vi "Setup TS DAC.vi"(8 "error in":errorcluster, 11 "HTS Test Stand in":refnum<class "HTS Test Stand.lvclass">) -> (0 "error out":errorcluster, 3 "HTS Test Stand out":refnum<class "HTS Test Stand.lvclass">)   [LabVIEW 2019, in "Test Stands.lvlib" / "HTS Test Stand.lvclass"]
uses:
  HTS Test Stand.lvclass
  C:/Users/wg/Documents/LV_Projects/test-stand/App/Generic Test Stand/Generic Test Stand.lvclass
  DAC/LNG Boiling/Heater Box Temperatures/DAC Heater Box Temperatures.lvclass
  C:/Users/wg/Documents/LV_Projects/test-stand/App/DAC/DAC.lvclass
  DAC/DAC.lvclass
  DAC/LNG Boiling/Shunt dU/DAC Shunt dU.lvclass
  DAC/LNG Boiling/Heater dU/DAC Heater dU.lvclass
  DAC/LNG Boiling/Heater Ctrl/DAC Heater Ctrl.lvclass
  DAC/DAC.lvclass/DAC.ctl
  Generic Test Stand/Generic Test Stand.lvclass/Generic Test Stand.ctl
  Generic Test Stand/Generic Test Stand.lvclass
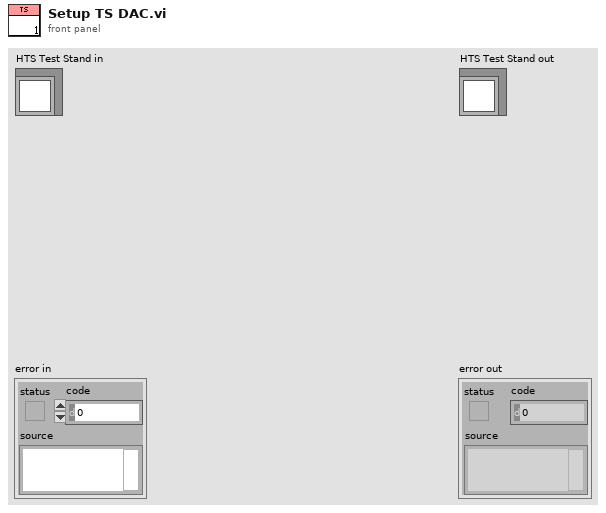
[diagram p1: front panel]
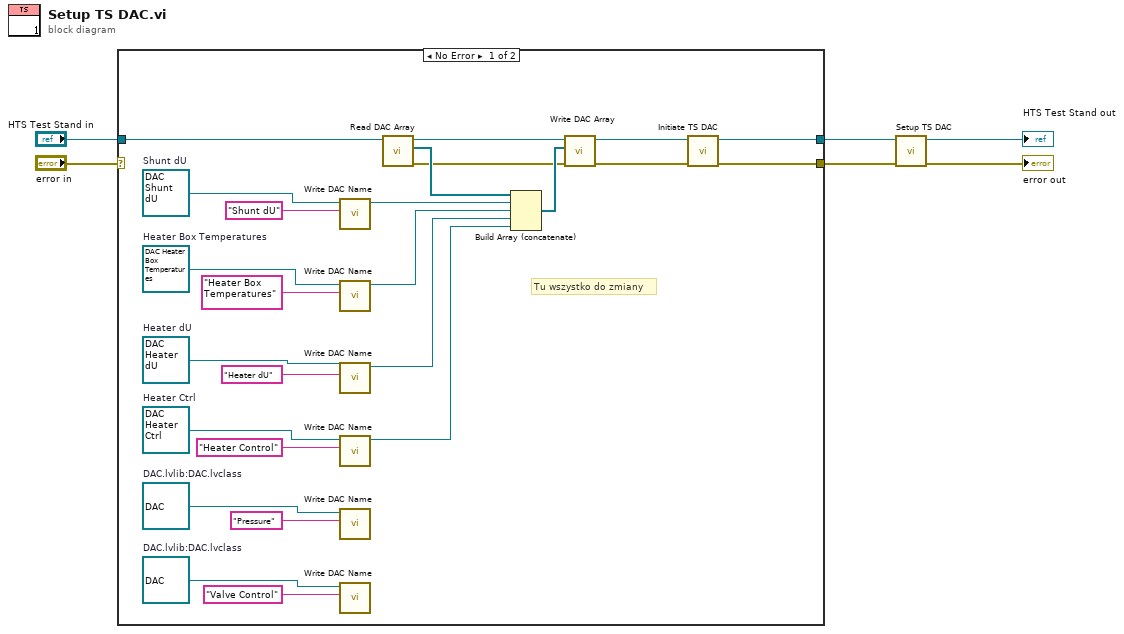
[diagram p0: block diagram]
diagram:
  n1 = case shown="No Error" "error in" {
    selector: "error in" -> [_ w32]
    tunnel: "HTS Test Stand in" -> [w26 w33]
    tunnel: [w8 w33] -> w2
    tunnel: [w7 w32] -> w1
    frame No Error {
      w11 = refnum<class "DAC Heater Ctrl.lvclass"> refnum  # Heater Ctrl
      w13 = refnum<class "DAC Heater dU.lvclass"> refnum  # Heater dU
      w15 = refnum<class "DAC Shunt dU.lvclass"> refnum  # Shunt dU
      w17 = refnum<class "DAC.lvclass"> refnum  # DAC.lvlib:DAC.lvclass
      w18 = refnum<class "DAC.lvclass"> refnum  # DAC.lvlib:DAC.lvclass
      w27 = refnum<class "DAC Heater Box Temperatures.lvclass"> refnum  # Heater Box Temperatures
      # "Tu wszystko do zmiany"
      n2 = call "Write DAC Name.vi"("DAC Name"="Shunt dU", "DAC in"=w15) -> ("DAC out"=w21:refnum<class "DAC Shunt dU.lvclass">)  [unwired: 8 in, 1 out]
      n3 = call "Write DAC Name.vi"("DAC Name"="Heater Box Temperatures", "DAC in"=w27) -> ("DAC out"=w20:refnum<class "DAC Heater Box Temperatures.lvclass">)  [unwired: 8 in, 1 out]
      n4 = call "Write DAC Name.vi"("DAC Name"="Heater dU", "DAC in"=w13) -> ("DAC out"=w14:refnum<class "DAC Heater dU.lvclass">)  [unwired: 8 in, 1 out]
      n5 = call "Write DAC Name.vi"("DAC Name"="Heater Control", "DAC in"=w11) -> ("DAC out"=w12:refnum<class "DAC Heater Ctrl.lvclass">)  [unwired: 8 in, 1 out]
      n6 = call "Write DAC Name.vi"("DAC Name"="Pressure", "DAC in"=w18) -> ()  [unwired: 8 in, 2 out]
      n7 = call "Write DAC Name.vi"("DAC Name"="Valve Control", "DAC in"=w17) -> ()  [unwired: 8 in, 2 out]
      n8 = call "Read DAC Array.vi"("Generic Test Stand in"=w26) -> ("error out"=w22:errorcluster, "DAC Array"=w25:refnum<class "DAC.lvclass">[], "Generic Test Stand out"=w24:refnum<class "HTS Test Stand.lvclass">)  [unwired: 8 in]
      n9 = Build Array (concatenate)(w25, w21, w20, w14, w12) -> (w23:refnum<class "DAC.lvclass">[])
      n10 = call "Write DAC Array.vi"("error in (no error)"=w22, "DAC Array"=w23, "Generic Test Stand in"=w24) -> ("error out"=w9:errorcluster, "Generic Test Stand out"=w10:refnum<class "HTS Test Stand.lvclass">)  [unwired: 7 in]
      n11 = call-dynamic "Initiate TS DAC.vi"("error in (no error)"=w9, "Generic Test Stand in"=w10) -> ("error out"=w7:errorcluster, "Generic Test Stand out"=w8:refnum<class "HTS Test Stand.lvclass">)  [unwired: 8 in]
    }
    frame Error {
    }
  }
  n12 = call-parent "Setup TS DAC.vi"("error in (no error)"=w1, "Generic Test Stand in"=w2) -> ("error out"=→"error out":errorcluster, "Generic Test Stand out"=→"HTS Test Stand out":refnum<class "HTS Test Stand.lvclass">)  [unwired: 8 in]
